vi "GDX_XYGraph.vi"() -> ()   [LabVIEW 2019]
panel:
  out "XY Graph":cluster{dbl[], dbl[]}[](graph)
  in  "stop":bool
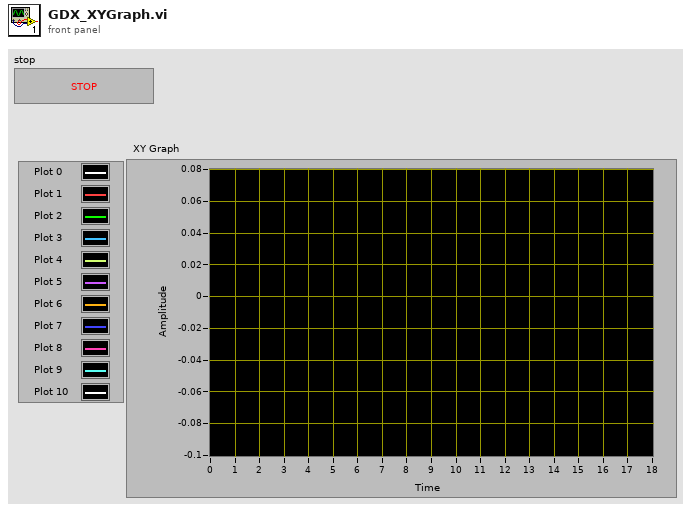
[diagram p1: front panel]
types:
  T1 = enum16{"Activate from Dialog Popup", "Activate All Channels", "Input On/Off Array", "Input Channel  Mask", "Burn Sensor Default Channels"}
  T2 = enum16{"Set Rate from Dialog Popup", "Default 1 Sample/Sec", "Input Sample Rate"}
  T3 = typedef "D2PIO_D2PIOCluster.ctl" = cluster{"Library Handle":i64, "Device List Handle":i64, "BT Device Handles":i64[], "USB Device Handles":i64[], "BT+USB Device Handles":i64[], "Measurement Tick":dbl[], "Ch Availability Mask":u32[]}
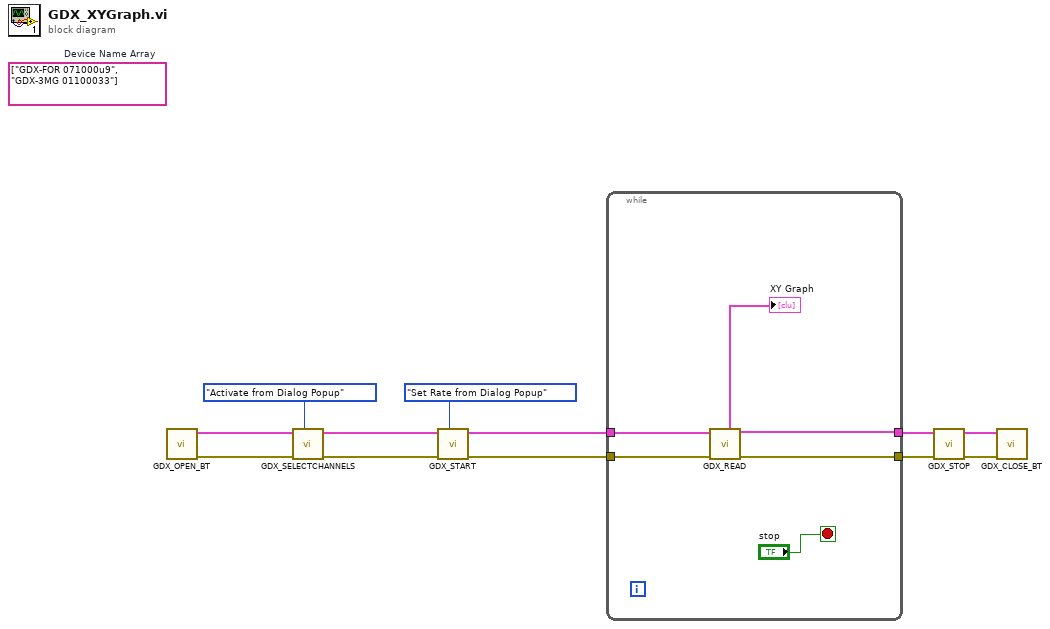
[diagram p0: block diagram]
diagram:
  (unwired) string[] ["GDX-FOR 071000u9", "GDX-3MG 01100033"]  # Device Name Array
  n1 = call <vilib>:"GDX_OPEN_BT.vi"() -> ("error out"=w6:errorcluster, "D2PIO Cluster Out"=w7:T3)  [unwired: 10 in]
  n2 = call <vilib>:"GDX_SELECTCHANNELS.vi"("Enum"=T1."Activate from Dialog Popup", "error in (no error)"=w6, "D2PIO Cluster In"=w7) -> ("error out"=w3:errorcluster, "D2PIO Cluster Out"=w4:T3)  [unwired: 7 in]
  n3 = call <vilib>:"GDX_START.vi"("Enum"=T2."Set Rate from Dialog Popup", "error in (no error)"=w3, "D2PIO Cluster In"=w4) -> ("error out"=w12:errorcluster, "D2PIO Cluster Out"=w11:T3)  [unwired: 5 in, 2 out]
  n4 = while {
    tunnel: w12 -> [w18]
    tunnel: w11 -> [w16]
    tunnel: [w13] -> w10
    tunnel: [w14] -> w5
    stop <- "stop" stop-if-true
    n5 = call <vilib>:"GDX_READ.vi"("error in (no error)"=w18, "D2PIO Cluster In"=w16) -> ("error out"=w14:errorcluster, "D2PIO Cluster Out"=w13:T3, "XY Graph Data"=→"XY Graph":cluster{dbl[], dbl[]}[])  [unwired: 4 in, 3 out]
  }
  n6 = call <vilib>:"GDX_STOP.vi"("error in (no error)"=w5, "D2PIO Cluster In"=w10) -> ("error out"=w8:errorcluster, "D2PIO Cluster Out"=w9:T3)  [unwired: 8 in]
  n7 = call <vilib>:"GDX_CLOSE_BT.vi"("error in (no error)"=w8, "D2PIO Cluster In"=w9) -> ()  [unwired: 8 in, 2 out]
